vi "XML Parser.vi"(8 "error in (no error)":errorcluster, 9 "Path 3":path=path "C:/Users/Staff1/Desktop/Raw_Data.txt", 10 "Path 2":path=path "C:/Users/Staff1/Desktop/Data_With_Header.txt", 11 "Path":path) -> (0 "error out":errorcluster)   [LabVIEW 2017]
uses:
  <vilib>/xml/Load XML File.vi
  <vilib>/xml/Close Reference(Node).vi
  <vilib>/xml/NI_XML.lvlib
panel:
  out "Value Out":string
  out "Parse Error 1":string
  out "Address Out":string
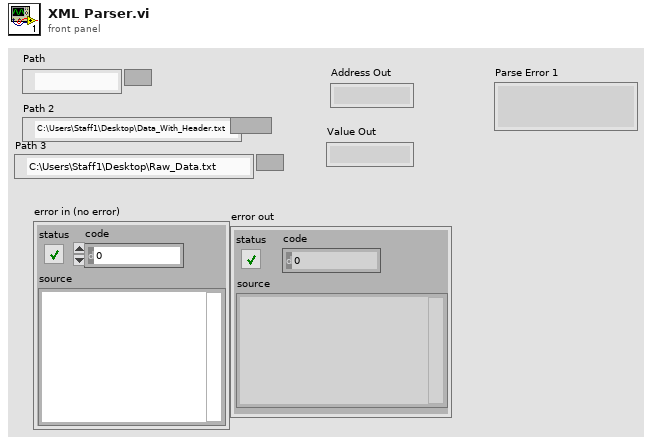
[diagram p1: front panel]
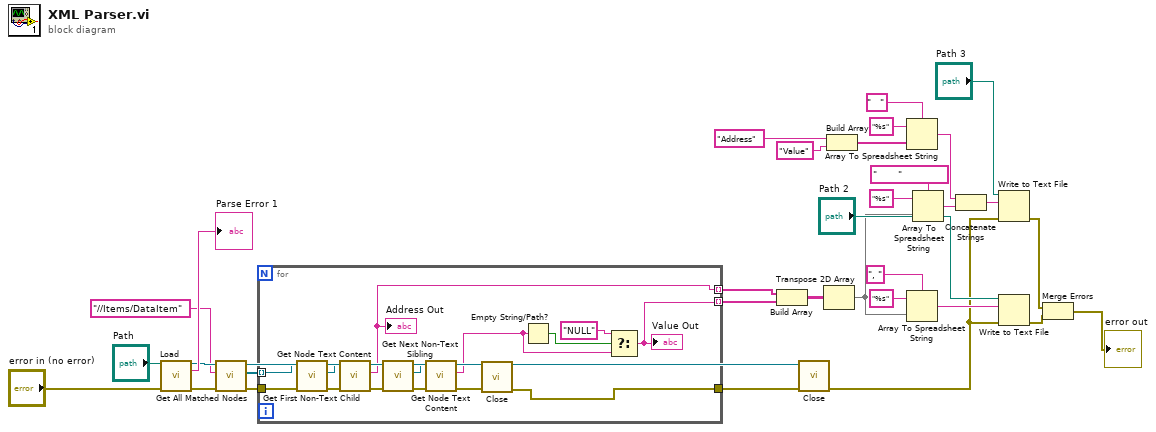
[diagram p0: block diagram]
diagram:
  n1 = call-poly <vilib>:"Load.vi"("path to XML document"="Path", "error in (no error)"="error in (no error)") -> ("DOM document out"=w30:refnum<k20>, "parse errors"=→"Parse Error 1":string, "error out"=w28:errorcluster)  [unwired: 11 in]
  n2 = call <vilib>:"Get All Matched Nodes.vi"("error in (no error)"=w28, "XPath expression"="//Items/DataItem", "node in"=w30) -> ("error out"=w26:errorcluster, "node result array"=w27:refnum<k20>[], "node out"=w1:refnum<k20>)  [unwired: 6 in]
  n3 = for {
    tunnel: w27 -> [w43] mode=indexing
    tunnel: w26 -> [w42]
    tunnel: [w38] -> w24 mode=indexing
    tunnel: [w37] -> w25 mode=indexing
    tunnel: [w34] -> w3
    n4 = call <vilib>:"Get First Non-Text Child.vi"("error in (no error)"=w42, "node in"=w43) -> ("error out"=w44:errorcluster, "child node"=w45:refnum<k20>)  [unwired: 6 in, 2 out]
    n5 = call <vilib>:"Get Node Text Content.vi"("error in (no error)"=w44, "node in"=w45) -> ("error out"=w48:errorcluster, "node text"=w37:string, "node out"=w49:refnum<k20>)  [unwired: 7 in]
    "Address Out" <- w37
    n6 = call <vilib>:"Get Next Non-Text Sibling.vi"("error in (no error)"=w48, "node in"=w49) -> ("error out"=w46:errorcluster, "sibling node"=w47:refnum<k20>)  [unwired: 6 in, 2 out]
    n7 = call <vilib>:"Get Node Text Content.vi"("error in (no error)"=w46, "node in"=w47) -> ("error out"=w35:errorcluster, "node text"=w39:string, "node out"=w36:refnum<k20>)  [unwired: 7 in]
    n8 = call-poly <vilib>:"Close.vi"("error in (no error)"=w35, "node"=w36) -> ("error out"=w34:errorcluster)  [unwired: 7 in]
    n9 = Empty String/Path?(string/path=w39) -> (empty?=w41:bool)
    n10 = Select(t="NULL", s=w41, f=w39) -> (s? t:f=w38:string)
    "Value Out" <- w38
  }
  n11 = Build Array(w25, w24) -> (w21:string[][])
  n12 = call-poly <vilib>:"Close.vi"("error in (no error)"=w3, "node"=w1) -> ("error out"=w2:errorcluster)  [unwired: 7 in]
  n13 = Transpose 2D Array(2D array=w21) -> (transposed array=w8:string[][])
  n14 = Build Array("Address", "Value") -> (w16:string[])
  n15 = Array To Spreadsheet String(delimiter (Tab)="   ", array=w16, 3:"%s") -> (spreadsheet string=w14:string)
  n16 = Array To Spreadsheet String(delimiter (Tab)=", ", array=w8, 3:"%s") -> (spreadsheet string=w7:string)
  n17 = Array To Spreadsheet String(delimiter (Tab)="       ", array=w8, 3:"%s") -> (spreadsheet string=w12:string)
  n18 = Concatenate Strings(w14, w12) -> (w15:string)
  n19 = Write to Text File(file (use dialog)="Path 3", text=w15, error in=w2) -> (error out=w5:errorcluster)  [unwired: 1 in, 2 out]
  n20 = Write to Text File(file (use dialog)="Path 2", text=w7, error in=w2) -> (error out=w6:errorcluster)  [unwired: 1 in, 2 out]
  n21 = Merge Errors(w5, w6) -> (→"error out":errorcluster)
